vi "partBreal.vi"() -> ()   [LabVIEW 2010]
uses:
  <vilib>/Utility/file.llb/Write To Spreadsheet File (DBL).vi
  <vilib>/Analysis/NI_AALBase.lvlib
panel:
  in  "mode (0)":i16
  out "Numeric 3":dbl
  in  "Waittemp":dbl format="%.2f"
  in  "Steptemp":dbl format="%.2f"
  in  "Stopfreq":dbl format="%.2f"
  in  "Startfreq":dbl format="%.2f"
  in  "Stoptemp":dbl format="%.2f"
  in  "Starttemp":dbl format="%.2f"
  out "Numeric 2":dbl format="%.2f"
  in  "Step 2":dbl format="%.2f"
  in  "Stop 2":dbl format="%.2f"
  in  "Start 2":dbl format="%.2f"
  out "data":string
  out "Numeric":dbl format="%.2f"
  out "XY Graph 2":cluster{dbl[], dbl[]}(graph)
  out "XY Graph":cluster{dbl[], dbl[]}(graph)
  in  "Path":path
  out "error out 2":errorcluster
  in  "Wait/s":dbl format="%.2f"
  in  "Stepfreq":dbl format="%.2f"
  in  "error in (no error)":errorcluster
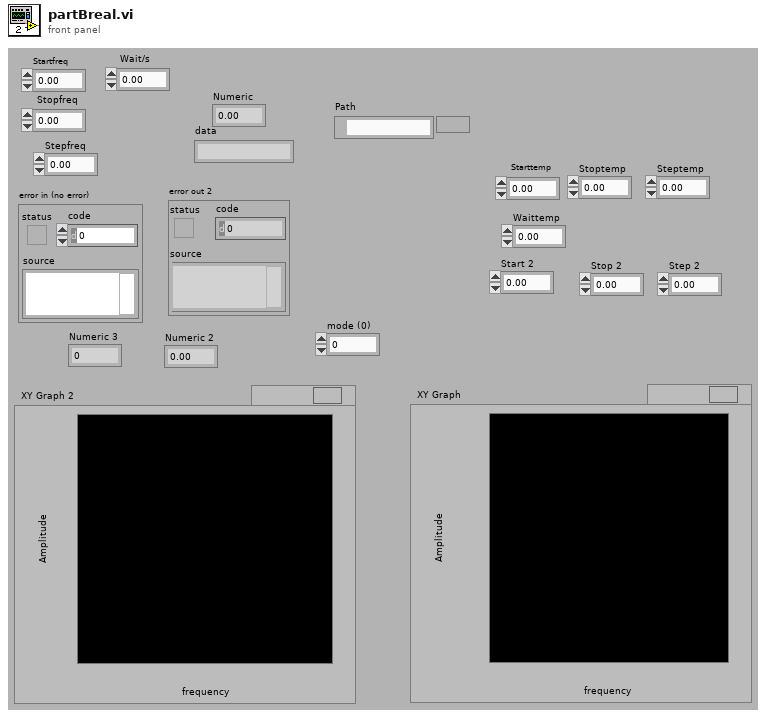
[diagram p1: front panel]
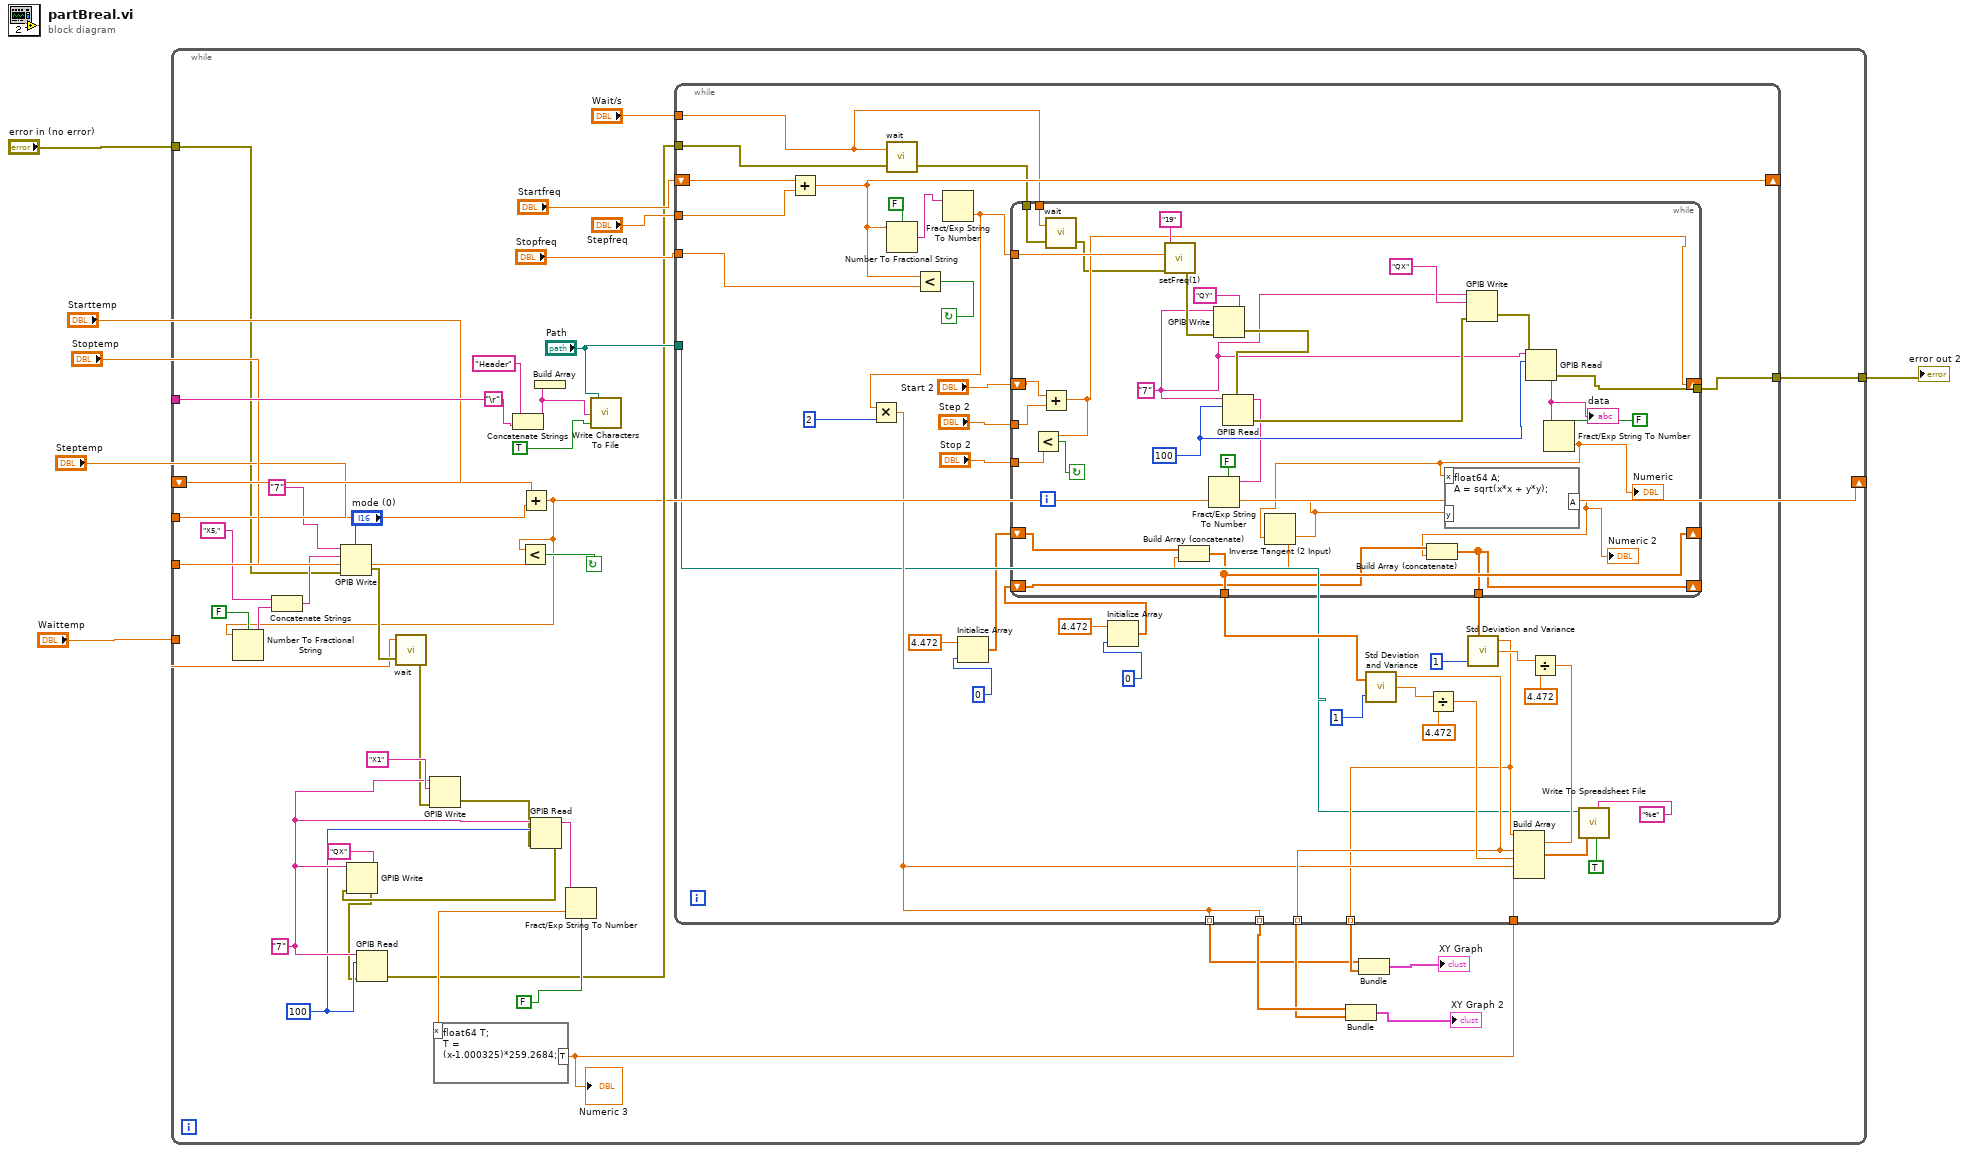
[diagram p0: block diagram]
diagram:
  n1 = while {
    tunnel: "\r" -> [w47]
    tunnel: [w37] -> w6
    shift-right: [w9] -> _
    shift-left: "Starttemp" -> [w34]
    tunnel: "Stoptemp" -> [w32]
    tunnel: "Steptemp" -> [w33]
    tunnel: "Waittemp" -> [w12]
    tunnel: "error in (no error)" -> [w11]
    stop <- w31 continue-if-true
    w26 = 100
    w28 = "7"
    n2 = Concatenate Strings("Header", w47) -> (w45:string)
    n3 = Add(x=w34, y=w33) -> (x+y=w9:dbl)
    n4 = Number To Fractional String(use system decimal point (T)=FALSE, number=w9) -> (F-format string=w16:string)  [unwired: 2 in]
    n5 = Concatenate Strings("X5,", w16) -> (w14:string)
    n6 = GPIB Write(0:"7", 1:w14, 2:"mode (0)", 3:w11) -> (6:w17:errorcluster)  [unwired: 1 in, 1 out]
    n7 = call "wait.vi"("error in"=w17, "Wartezeit in Sek"=w12) -> ("error out"=w13:errorcluster)  [unwired: 1 in]
    n8 = GPIB Write(0:w28, 1:"X1", 3:w13) -> (6:w25:errorcluster)  [unwired: 2 in, 1 out]
    n9 = Less?(x=w9, y=w32) -> (x < y?=w31:bool)
    n10 = GPIB Read(0:w28, 1:w26, 3:w25) -> (5:w23:string, 7:w22:errorcluster)  [unwired: 2 in, 1 out]
    n11 = GPIB Write(0:w28, 1:"QX", 3:w22) -> (6:w21:errorcluster)  [unwired: 2 in, 1 out]
    n12 = GPIB Read(0:w28, 1:w26, 3:w21) -> (7:w10:errorcluster)  [unwired: 2 in, 2 out]
    n13 = Build Array(w45) -> ()  [unwired: 1 out]
    n14 = Fract/Exp String To Number(use system decimal point (T)=FALSE, string=w23) -> (number=w24:dbl)  [unwired: 2 in, 1 out]
    n15 = formula code="float64 T;\nT = (x-1.000325)*259.2684;"("x"=w24) -> ("T"=w8:dbl)
    "Numeric 3" <- w8
    n16 = call <vilib>:"Write Characters To File.vi"("append to file? (new file:F)"=TRUE, "character string"=w45, "file path (dialog if empty)"="Path") -> ()  [unwired: 2 in, 1 out]
    n17 = while {
      tunnel: w10 -> [w84]
      shift-right: [w85] -> _
      shift-left: "Startfreq" -> [w88]
      tunnel: "Stepfreq" -> [w90]
      tunnel: "Stopfreq" -> [w89]
      tunnel: "Wait/s" -> [w61]
      tunnel: "Path" -> [w58]
      tunnel: [w79] -> w37
      tunnel: [w65] -> w41 mode=indexing
      tunnel: [w66] -> w40 mode=indexing
      tunnel: [w65] -> w38 mode=indexing
      tunnel: [w63] -> w39 mode=indexing
      tunnel: w8 -> [w51]
      stop <- w87 continue-if-true
      n18 = Add(x=w88, y=w90) -> (x+y=w85:dbl)
      n19 = call "wait.vi"("error in"=w84, "Wartezeit in Sek"=w61) -> ("error out"=w83:errorcluster)  [unwired: 1 in]
      n20 = Number To Fractional String(use system decimal point (T)=FALSE, number=w85) -> (F-format string=w82:string)  [unwired: 2 in]
      n21 = Less?(x=w85, y=w89) -> (x < y?=w87:bool)
      n22 = Fract/Exp String To Number(string=w82) -> (number=w75:dbl)  [unwired: 3 in, 1 out]
      n23 = Multiply(x=w75, y=2) -> (x*y=w65:dbl)
      n24 = Initialize Array(4.472, 0) -> (w55:dbl[])
      n25 = Initialize Array(4.472, 0) -> (w52:dbl[])
      n26 = while {
        tunnel: w83 -> [w99]
        tunnel: w75 -> [w117]
        tunnel: [w112] -> w79
        tunnel: "Step 2" -> [w105]
        tunnel: "Stop 2" -> [w104]
        tunnel: [w93] -> w74
        tunnel: [w95] -> w68
        shift-right: [w101] -> _
        shift-left: "Start 2" -> [w102]
        tunnel: w61 -> [w100]
        shift-right: [w95] -> _
        shift-left: w55 -> [w96]
        shift-right: [w93] -> _
        shift-left: w52 -> [w94]
        stop <- w103 continue-if-true
        w111 = 100
        w113 = "7"
        n27 = Add(x=w102, y=w105) -> (x+y=w101:dbl)
        n28 = Less?(x=w101, y=w104) -> (x < y?=w103:bool)
        n29 = call "wait.vi"("error in"=w99, "Wartezeit in Sek"=w100) -> ("error out"=w98:errorcluster)  [unwired: 1 in]
        n30 = call "setFreq(1).vi"("error in"=w98, "Frequenz in Hz"=w117, "address string"="19") -> ("error out"=w118:errorcluster)  [unwired: 3 in]
        n31 = GPIB Write(0:w113, 1:"QY", 3:w118) -> (6:w119:errorcluster)  [unwired: 2 in, 1 out]
        n32 = GPIB Read(0:w113, 1:w111, 3:w119) -> (5:w109:string, 7:w115:errorcluster)  [unwired: 2 in, 1 out]
        n33 = Fract/Exp String To Number(use system decimal point (T)=FALSE, string=w109) -> (number=w110:dbl)  [unwired: 2 in, 1 out]
        n34 = GPIB Write(0:w113, 1:"QX", 3:w115) -> (6:w114:errorcluster)  [unwired: 2 in, 1 out]
        n35 = GPIB Read(0:w113, 1:w111, 3:w114) -> (5:w107:string, 7:w112:errorcluster)  [unwired: 2 in, 1 out]
        "data" <- w107
        n36 = Fract/Exp String To Number(use system decimal point (T)=FALSE, string=w107) -> (number=w108:dbl)  [unwired: 2 in, 1 out]
        "Numeric" <- w108
        n37 = Inverse Tangent (2 Input)(1:w108, 2:w110) -> (0:w97:dbl)
        n38 = Build Array (concatenate)(w96, w97) -> (w95:dbl[])
        n39 = formula code="float64 A;\nA = sqrt(x*x + y*y);"("x"=w108, "y"=w110) -> ("A"=w92:dbl)
        "Numeric 2" <- w92
        n40 = Build Array (concatenate)(w94, w92) -> (w93:dbl[])
      }
      n41 = call <vilib>:"Std Deviation and Variance.vi"("X"=w68, "Weighting (Sample)"=1) -> ("mean"=w66:dbl, "standard deviation"=w70:dbl)  [unwired: 1 out]
      n42 = Divide(x=w70, y=4.472) -> (x/y=w67:dbl)
      n43 = call <vilib>:"Std Deviation and Variance.vi"("X"=w74, "Weighting (Sample)"=1) -> ("mean"=w63:dbl, "standard deviation"=w73:dbl)  [unwired: 1 out]
      n44 = Divide(x=w73, y=4.472) -> (x/y=w71:dbl)
      n45 = Build Array(w63, w71, w66, w67, w65, w51) -> (w64:dbl[])
      n46 = call-poly <vilib>:"Write To Spreadsheet File.vi"("format (%.3f)"="%e", "append to file? (new file:F)"=TRUE, "1D data"=w64, "file path (dialog if empty)"=w58) -> ()  [unwired: 4 in, 1 out]
    }
    n47 = Bundle(w41, w40) -> (→"XY Graph 2":cluster{dbl[], dbl[]})  [unwired: 1 in]
    n48 = Bundle(w38, w39) -> (→"XY Graph":cluster{dbl[], dbl[]})  [unwired: 1 in]
  }
  "error out 2" <- w6
